vi "随机正整数.vi"(11 "输入":dbl) -> (3 "输出":i32)   [LabVIEW 2012]
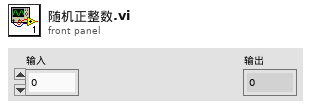
[diagram p1: front panel]
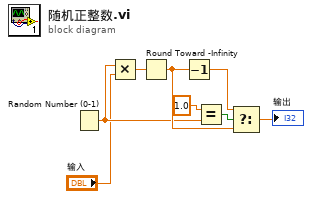
[diagram p0: block diagram]
diagram:
  n1 = Random Number (0-1)() -> (number: 0 to 1=w5:dbl)
  n2 = Multiply(x=w5, y="输入") -> (x*y=w3:dbl)
  n3 = Round Toward -Infinity(1:w3) -> (0:w8:dbl)
  n4 = Decrement(x=w8) -> (x-1=w7:dbl)
  n5 = Equal?(x=1.0, y=w5) -> (x = y?=w6:bool)
  n6 = Select(t=w7, s=w6, f=w8) -> (s? t:f=→"输出":dbl)
